vi "AddControl_Core.vi"(8 "error in (no error)":errorcluster, 9 "CtlRef":refnum<vi>, 10 "CtlName":string, 11 "ctlRef_Maps in":refnum<class "ctlRef_Maps.lvclass">) -> (0 "error out":errorcluster, 3 "ctlRef_Maps out":refnum<class "ctlRef_Maps.lvclass">)   [LabVIEW 2020, in "CtlReferences.lvlib" / "ctlRef_Maps.lvclass"]
uses:
  ctlRef_Maps.lvclass
  ctlRef_Maps.lvclass/ctlRef_Maps.ctl
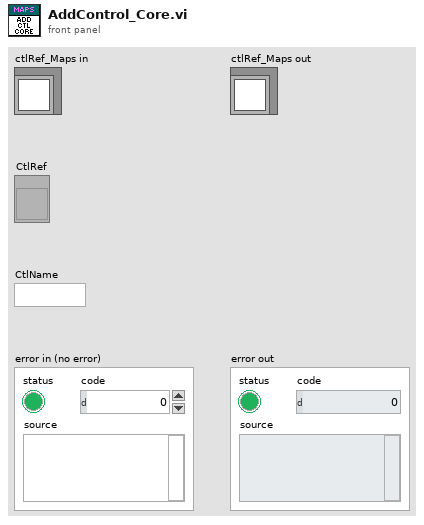
[diagram p1: front panel]
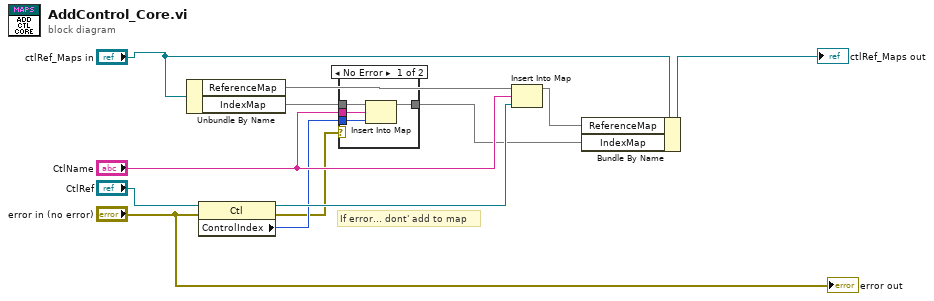
[diagram p0: block diagram]
diagram:
  # "If error... dont' add to map"
  n1 = Unbundle By Name("ctlRef_Maps in") -> ("ReferenceMap"=w11:map{string, refnum<vi>}, "IndexMap"=w8:map{string, i32})
  n2 = property class="Ctl"(reference="CtlRef", error in="error in (no error)") -> (reference out=w9:refnum<vi>, error out=w1:errorcluster, "ControlIndex"=w6:i32)
  n3 = case shown="No Error" w1 {
    tunnel: w8 -> [w16 w17]
    tunnel: "CtlName" -> [w15 _]
    tunnel: w6 -> [w14 _]
    tunnel: [w13 w17] -> w3
    frame No Error {
      n4 = Insert Into Map(map in=w16, key=w15, value=w14) -> (map out=w13:map{string, i32})  [unwired: 2 out]
    }
    frame Error {
    }
  }
  n5 = Insert Into Map(map in=w11, key="CtlName", value=w9) -> (map out=w4:map{string, refnum<vi>})  [unwired: 2 out]
  n6 = Bundle By Name(cluster="ctlRef_Maps in", "ReferenceMap"=w4, "IndexMap"=w3) -> (→"ctlRef_Maps out":refnum<class "ctlRef_Maps.lvclass">)
  "error out" <- "error in (no error)"
